vi "Initialize Core.vi"(8 "Error In":errorcluster, 11 "TDMS Log In":refnum<class "TDMS Logger.lvclass">) -> (0 "Error Out":errorcluster, 3 "TDMS Log Out":refnum<class "TDMS Logger.lvclass">)   [LabVIEW 2014, in "TDMS Logger.lvlib" / "TDMS Logger.lvclass"]
uses:
  TDMS Logger.lvclass
  TDMS Logger.lvclass/TDMS Logger.ctl
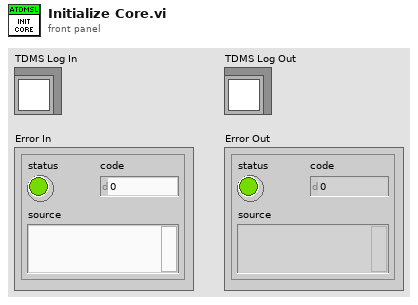
[diagram p1: front panel]
types:
  T1 = enum16{"open", "open or create", "create or replace", "create", "open (read-only)"}
  T2 = typedef "TDMS Logger.lvlib/TDMS Logger.lvclass/Multiple Files Action.ctl" = enum16{"Seperate based on size", "Seperate based on time", "Single file"}
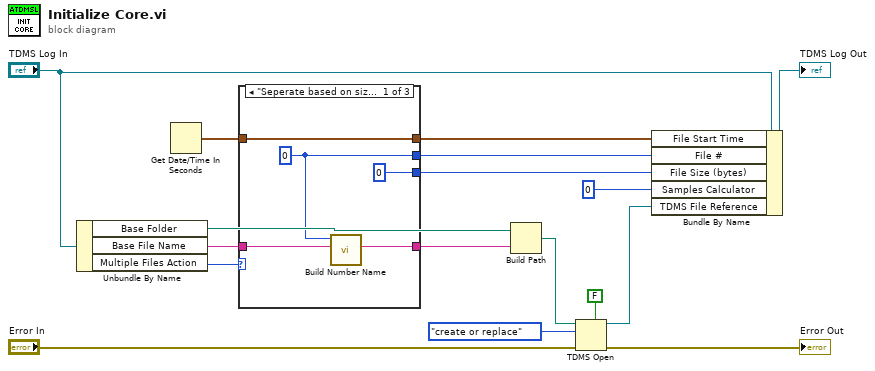
[diagram p0: block diagram]
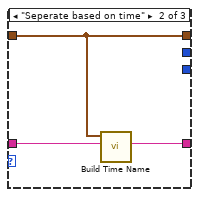
[diagram p2: hidden frame]
diagram:
  n1 = Unbundle By Name("TDMS Log In") -> ("Base Folder"=w2:path, "Base File Name"=w11:string, "Multiple Files Action"=w10:T2)
  n2 = Get Date/Time In Seconds() -> (seconds since 1Jan1904=w1:timestamp)
  n3 = case shown="\"Seperate based on size\", Default" w10 {
    tunnel: w11 -> [w22 w25 w27]
    tunnel: [w21 w24 w27] -> w12
    tunnel: [w20 _ _] -> w14
    tunnel: [w18 w23 w26] -> w15
    tunnel: [u64 0 ("File Size (bytes)") _ _] -> w16
    tunnel: w1 -> [w18 w23 w26]
    frame "Seperate based on size", Default {
      w20 = u32 0 ("File #")
      n4 = call "Build Number Name.vi"("Base File Name"=w22, "File #"=w20) -> ("Numbered Name"=w21:string)  [unwired: 9 in]
    }
    frame "Seperate based on time" {
      n5 = call "Build Time Name.vi"("Base File Name"=w25, "Timestamp"=w23) -> ("Time Name"=w24:string)  [unwired: 9 in]
    }
    frame "Single file" {
    }
  }
  n6 = Build Path(base path=w2, name or relative path=w12) -> (appended path=w3:path)
  n7 = TDMS Open(5:FALSE ("create index file? (T)"), 8:"Error In", 10:T1."create or replace" ("operation (0:open)"), 11:w3) -> (0:→"Error Out":errorcluster, 3:w8:refnum<k34>)  [unwired: 3 in]
  n8 = Bundle By Name(cluster="TDMS Log In", "File Start Time"=w15, "File #"=w14, "File Size (bytes)"=w16, "Samples Calculator"=u32 0, "TDMS File Reference"=w8) -> (→"TDMS Log Out":refnum<class "TDMS Logger.lvclass">)
